vi "Write Class Data.vi"(8 "error in (no error)":errorcluster, 9 "Load Failure":string[](array[string]), 10 "Load Success":string[](array[string]), 11 "PPL Class Test Data in":refnum<class "PPL Class Test Data.lvclass">) -> (0 "error out":errorcluster, 3 "PPL Class Test Data out":refnum<class "PPL Class Test Data.lvclass">)   [LabVIEW 2019, in "ProjectBuilder.lvlib" / "PPL Class Test Data.lvclass"]
doc: "Read success and fail string arrays from the private data."
uses:
  PPL Class Test Data.lvclass
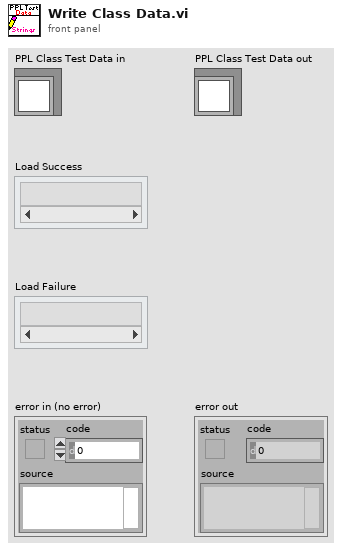
[diagram p1: front panel]
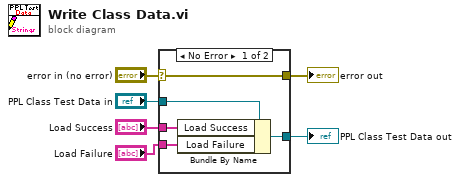
[diagram p0: block diagram]
diagram:
  n1 = case shown="No Error" "error in (no error)" {
    selector: "error in (no error)" -> [w11 w12]
    tunnel: [w11 w12] -> w5
    tunnel: [w9 w13] -> w3
    tunnel: "PPL Class Test Data in" -> [w10 w13]
    tunnel: "Load Success" -> [w8 _]
    tunnel: "Load Failure" -> [w7 _]
    frame No Error {
      n2 = Bundle By Name(cluster=w10, "Load Success"=w8, "Load Failure"=w7) -> (w9:refnum<class "PPL Class Test Data.lvclass">)
    }
    frame Error {
    }
  }
  "error out" <- w5
  "PPL Class Test Data out" <- w3
